vi "Remove Plugin.vi"(7 "name":string, 8 "error in (no error)":errorcluster, 11 "dsf refnum":T1) -> (0 "error out":errorcluster, 2 "exists?":bool, 3 "dsf refnum out":T1)   [LabVIEW 2017, in "DSF Configuration API.lvlib"]
doc: "Removes a section from the configuration data identified by <B>dsf refnum</B>."
uses:
  DSF Configuration API.lvlib
  Controls/DSF Config Data RefNum.ctl
  Private/Session/Typecast Refnum to Queue.vi
  Private/Session/Typecast Queue to Refnum.vi
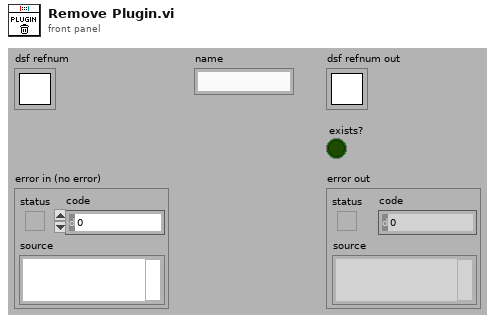
[diagram p1: front panel]
types:
  T1 = typedef "DSF Configuration API.lvlib/DSF Config Data RefNum.ctl" = refnum<k1>
  T2 = typedef "DSF Configuration API.lvlib/DSF Configuration Reference.ctl" = refnum<data-value>
  T3 = typedef "DSF Configuration API.lvlib/Config Data.ctl" = cluster{"dsf configuration":T4, "path":path, "dirty":bool}
  T4 = typedef "DSF Configuration API.lvlib/DSF Config.ctl" = cluster{"dsfversion":T5, "version":T5, "plugins":T6[], "groups":T9[], "transfers":T11[], "channels":T13[], "settings":T15[]}
  T5 = typedef "DSF Configuration API.lvlib/Version Info.ctl" = cluster{"major":u32, "minor":u32, "fix":u32, "build":string}
  T6 = typedef "DSF Configuration API.lvlib/DSF Plugin.ctl" = cluster{"id":string, "values":T7}
  T7 = typedef "DSF Configuration API.lvlib/DSF Plugin Info.ctl" = cluster{"type":string, "timing":T8, "group ids":string[], "settings id":string}
  T8 = typedef "DSF Configuration API.lvlib/DSF Timing Info.ctl" = cluster{"priority":i32, "decimation":i32, "offset":i32}
  T9 = typedef "DSF Configuration API.lvlib/DSF Group.ctl" = cluster{"id":string, "values":T10}
  T10 = typedef "DSF Configuration API.lvlib/DSF Group Info.ctl" = cluster{"direction":i32, "timing":T8, "transfer ids":string[], "settings id":string}
  T11 = typedef "DSF Configuration API.lvlib/DSF Transfer.ctl" = cluster{"id":string, "values":T12}
  T12 = typedef "DSF Configuration API.lvlib/DSF Transfer Info.ctl" = cluster{"byte order":i32, "channel ids":string[], "settings id":string}
  T13 = typedef "DSF Configuration API.lvlib/DSF Channel.ctl" = cluster{"id":string, "values":T14}
  T14 = typedef "DSF Configuration API.lvlib/DSF Channel Info.ctl" = cluster{"count":i32, "offset":i32, "data type":i32, "resource path":string, "settings id":string}
  T15 = typedef "DSF Configuration API.lvlib/DSF Settings.ctl" = cluster{"id":string, "values":T16}
  T16 = typedef "DSF Configuration API.lvlib/DSF Settings Info.ctl" = cluster{"key":string, "value":string}[]
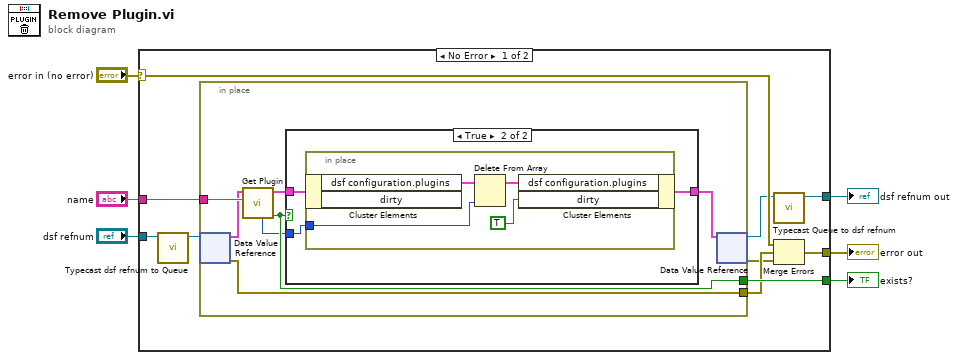
[diagram p0: block diagram]
diagram:
  n1 = case shown="No Error" "error in (no error)" {
    selector: "error in (no error)" -> [w14 w33]
    tunnel: [w9 w33] -> w1
    tunnel: [w15 w32] -> w3
    tunnel: "dsf refnum" -> [w16 w32]
    tunnel: "name" -> [w13 _]
    tunnel: [w12 _] -> w2
    frame No Error {
      n2 = call "Typecast dsf refnum to Queue.vi"("dsf refnum in"=w16) -> ("DSF Configuration Reference out"=w11:T2)  [unwired: 10 out]
      n3 = in-place {
        in-place-border: w13 -> [w23]
        in-place-border: [w22] -> w12
        in-place-border: [w17] -> w8
        n4 = in-place-dvr #1(w11) -> (w19:T3, w17:errorcluster)
        n5 = call "Get Plugin.vi"("id"=w23, "DSF Configuration in"=w19) -> ("exists?"=w22:bool, "DSF Configuration out"=w21:T3, "index"=w20:i32)  [unwired: 2 in, 5 out]
        n6 = case shown="True" w22 {
          tunnel: [w24 w27] -> w18
          tunnel: w20 -> [_ w26]
          tunnel: w21 -> [w24 w25]
          frame False {
          }
          frame True {
            n7 = in-place {
              in-place-border: w26 -> [w31]
              n8 = in-place-cluster #2(w25) -> ("dsf configuration.plugins"=w30:T6[])  [unwired: 1 out]
              n9 = Delete From Array(array=w30, index=w31) -> (array with subset deleted=w29:T6[])  [unwired: 1 in, 1 out]
              n10 = in-place-cluster #2("dsf configuration.plugins"=w29, "dirty"=TRUE) -> (w27:T3)
            }
          }
        }
        n11 = in-place-dvr #1(w18) -> (w10:T2, w7:errorcluster)
      }
      n12 = call "Typecast Queue to dsf refnum.vi"("DSF Configuration Reference in"=w10) -> ("dsf refnum out"=w15:T1)  [unwired: 10 out]
      n13 = Merge Errors(w14, w8, w7) -> (w9:errorcluster)
    }
    frame Error {
    }
  }
  "error out" <- w1
  "exists?" <- w2
  "dsf refnum out" <- w3
